vi "REGISTER (Async).vi"(0 "WAMP Client in":refnum<class "WAMP Client.lvclass">, 1 "Options":string, 5 "Procedure URI":string, 7 "INVOCATION event":refnum<user-event>, 9 "REGISTERED or ERROR event":refnum<user-event>, 11 "error in (no error)":errorcluster) -> (4 "WAMP Client out":refnum<class "WAMP Client.lvclass">, 15 "error out":errorcluster)   [LabVIEW 2020, in "WAMP Client.lvclass"]
uses:
  <userlib>/lvwamp/WAMP Client/WAMP Client.lvclass
  <userlib>/lvwamp/WAMP Client/WAMP Client.lvclass/WAMP Client.ctl
  <userlib>/lvwamp/WAMP Client/TypeDef/WAMP Error Payload.ctl
  <userlib>/lvwamp/WAMP Client/TypeDef/REGISTERED or ERROR payload.ctl
  <userlib>/lvwamp/WAMP Client/TypeDef/INVOCATION payload.ctl
  <userlib>/lvwamp/WAMP Client/TypeDef/REGISTER Request Data.ctl
  <userlib>/lvwamp/WAMP Client/TypeDef/Internal Message Type.ctl
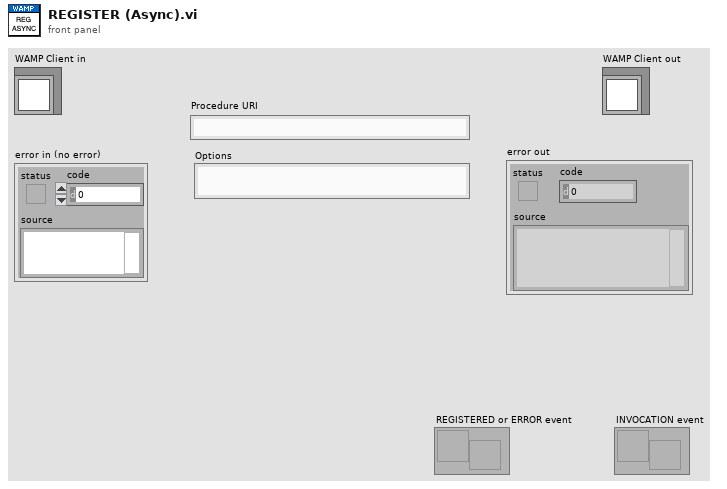
[diagram p1: front panel]
types:
  T1 = typedef "WAMP Client.lvclass/Internal Message Type.ctl" = enum16{"Subscribe", "Handle Subscribed", "Handle Event", "Unsubscribe", "Handle Unsubscribed", "Publish", "Handled Published", "Goodbye", "Handle Goodbye", "Call", "Handle Result", "Register", "Handle Registered", "Unregister", "Handle Unregistered", "Handle Invocation", "Yield"}
  T2 = typedef "WAMP Client.lvclass/REGISTER Request Data.ctl" = cluster{"Procedure URI":string, "Options":string, "REGISTERED or ERROR event":refnum<user-event>, "INVOCATION event":refnum<user-event>}
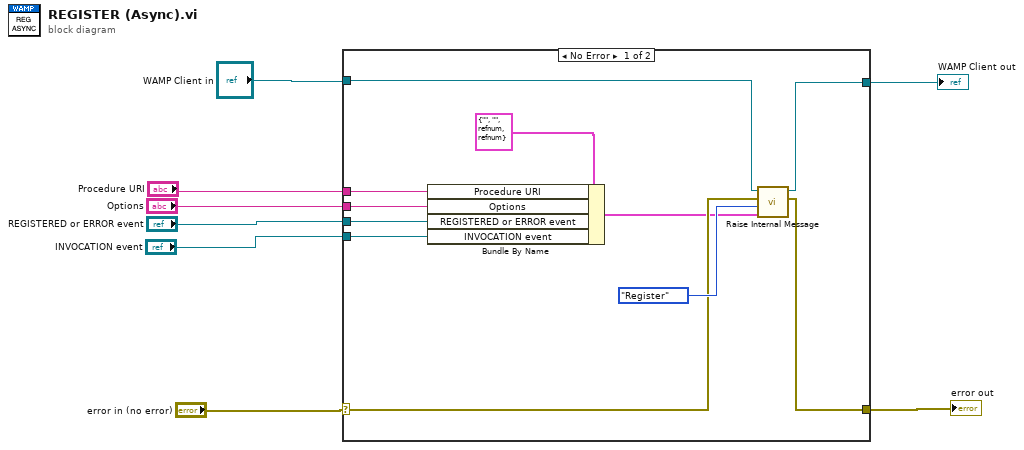
[diagram p0: block diagram]
diagram:
  n1 = case shown="No Error" "error in (no error)" {
    selector: "error in (no error)" -> [w11 w21]
    tunnel: [w9 w21] -> w7
    tunnel: [w13 w20] -> w5
    tunnel: "WAMP Client in" -> [w14 w20]
    tunnel: "Procedure URI" -> [w18 _]
    tunnel: "Options" -> [w17 _]
    tunnel: "REGISTERED or ERROR event" -> [w16 _]
    tunnel: "INVOCATION event" -> [w15 _]
    frame No Error {
      n2 = Bundle By Name(cluster=T2 {"Procedure URI"="", "Options"="", "REGISTERED or ERROR event"=refnum, "INVOCATION event"=refnum} ("REGISTER request data"), "Procedure URI"=w18, "Options"=w17, "REGISTERED or ERROR event"=w16, "INVOCATION event"=w15) -> (w10:T2)
      n3 = call-dynamic "Raise Internal Message.vi"("Variant"=w10, "Internal Message Type"=Internal_Message_Type."Register", "error in (no error)"=w11, "WAMP Client in"=w14) -> ("error out"=w9:errorcluster, "WAMP Client out"=w13:refnum<class "WAMP Client.lvclass">)  [unwired: 6 in]
    }
    frame Error {
    }
  }
  "error out" <- w7
  "WAMP Client out" <- w5
